vi "SecondsToTime.vi"(1 "Seconds":dbl format="%.2f") -> (0 "Time":string)   [LabVIEW 2009]
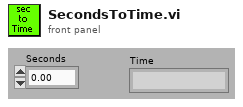
[diagram p1: front panel]
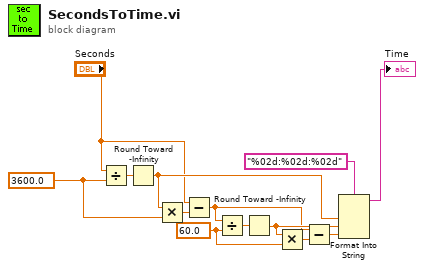
[diagram p0: block diagram]
diagram:
  w7 = 60.0 ("y")
  w3 = 3600.0 ("y")
  n1 = Divide(x="Seconds", y=w3) -> (x/y=w2:dbl)
  n2 = Round Toward -Infinity(1:w2) -> (0:w11:dbl)
  n3 = Multiply(x=w11, y=w3) -> (x*y=w4:dbl)
  n4 = Subtract(x="Seconds", y=w4) -> (x-y=w8:dbl)
  n5 = Divide(x=w8, y=w7) -> (x/y=w1:dbl)
  n6 = Round Toward -Infinity(1:w1) -> (0:w10:dbl)
  n7 = Multiply(x=w10, y=w7) -> (x*y=w6:dbl)
  n8 = Subtract(x=w8, y=w6) -> (x-y=w9:dbl)
  n9 = Format Into String(format string="%02d:%02d:%02d", w11, w10, w9) -> (resulting string=→"Time":string)  [unwired: 2 in, 1 out]
